vi "Process Calculation Results.vi"(8 "error in (no error)":errorcluster, 10 "Calculation Results":T1, 11 "CPU FFT Calculator in":refnum<class "CPU FFT Calculator.lvclass">) -> (0 "error out":errorcluster, 3 "CPU FFT Calculator out":refnum<class "CPU FFT Calculator.lvclass">)   [LabVIEW 2020, in "CPU FFT Calculator.lvlib" / "CPU FFT Calculator.lvclass"]
uses:
  CPU FFT Calculator.lvclass
  C:/Users/natan/Documents/G2CPU-Performance-Demo/Calculation Worker/Calculation Worker/Calculation Worker.lvclass
  C:/Program Files/National Instruments/LabVIEW 2026/vi.lib/ActorFramework/Actor/Actor.lvclass
  CPU Calculation Results.ctl
  CPU Metrics.ctl
  CPU FFT Calculator.lvclass/CPU FFT Calculator.ctl
  <vilib>/ActorFramework/Actor/Actor.lvclass/Actor.ctl
  Application Manager/Application Manager Messages/Update CPU UI Components Msg/Update CPU UI Components Msg.lvclass/Update CPU UI Components Msg.ctl
  <vilib>/ActorFramework/Message Enqueuer/Message Enqueuer.lvclass/Message Enqueuer.ctl
  Application Manager/Application Manager Messages/Update CPU Graph Msg/Update CPU Graph Msg.lvclass/Update CPU Graph Msg.ctl
  <vilib>/ActorFramework/Message Enqueuer/Enqueue.vi
  Application Manager/Application Manager Messages/Update CPU UI Components Msg/Update CPU UI Components Msg.lvclass
  C:/Program Files/National Instruments/LabVIEW 2026/vi.lib/ActorFramework/Message/Message.lvclass
  Application Manager/Application Manager Messages/Update CPU Graph Msg/Update CPU Graph Msg.lvclass
  <vilib>/ActorFramework/Message Priority Queue/Priority Enqueue.vi
  Simple UI/Simple UI/Simple UI.lvclass
  <vilib>/ActorFramework/Actor/Actor.lvclass
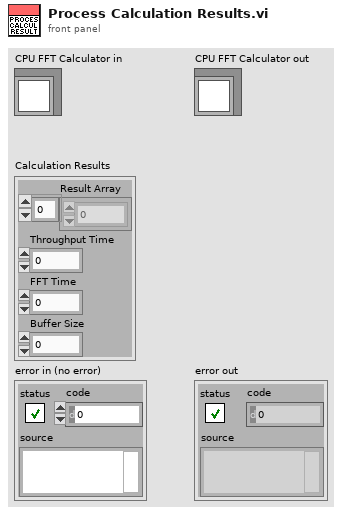
[diagram p1: front panel]
types:
  T1 = typedef "CPU FFT Calculator.lvlib/CPU FFT Calculator.lvclass/CPU Calculation Results.ctl" = cluster{"Result Array":sgl[], "Throughput Time":dbl, "FFT Time":dbl, "Buffer Size":i32}
  T2 = typedef "Simple UI.lvlib/Simple UI.lvclass/CPU Metrics.ctl" = cluster{"FFT Time":dbl, "Throughput":dbl, "Queue Depth":u64, "Elapsed Time":dbl}
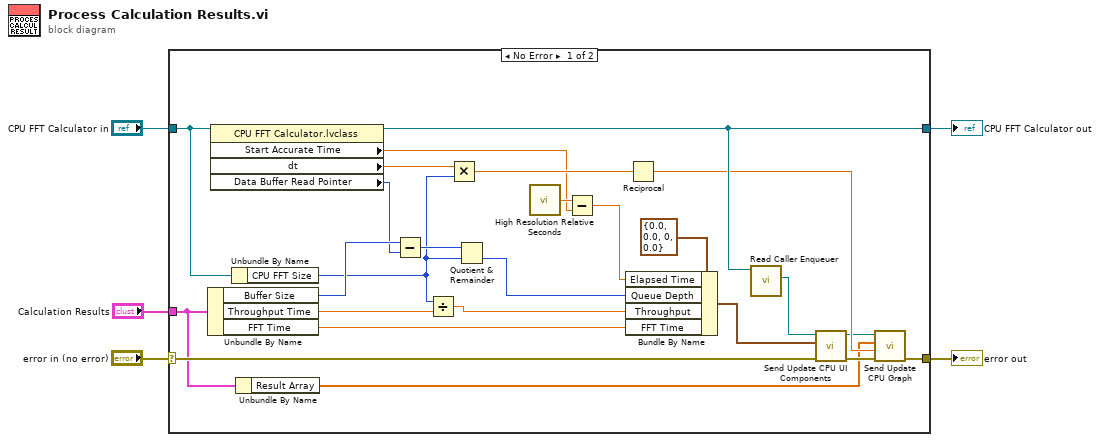
[diagram p0: block diagram]
diagram:
  n1 = case shown="No Error" "error in (no error)" {
    selector: "error in (no error)" -> [w24 w32]
    tunnel: [w16 w32] -> w4
    tunnel: [w22 w31] -> w2
    tunnel: "CPU FFT Calculator in" -> [w26 w31]
    tunnel: "Calculation Results" -> [w12 _]
    frame No Error {
      n2 = Unbundle By Name(w12) -> ("Buffer Size"=w21:i32, "Throughput Time"=w28:dbl, "FFT Time"=w29:dbl)
      n3 = property class="CPU FFT Calculator.lvclass"(reference=w26) -> (reference out=w22:refnum<class "CPU FFT Calculator.lvclass">, "Start Accurate Time"=w7:dbl, "dt"=w15:dbl, "Data Buffer Read Pointer"=w20:u64)  [unwired: 1 in, 1 out]
      n4 = Unbundle By Name(w26) -> ("CPU FFT Size"=w9:u64)
      n5 = Unbundle By Name(w12) -> ("Result Array"=w11:sgl[])
      n6 = Subtract(x=w21, y=w20) -> (x-y=w19:u64)
      n7 = Divide(x=w9, y=w28) -> (x/y=w27:dbl)
      n8 = Multiply(x=w15, y=w9) -> (x*y=w10:dbl)
      n9 = Quotient & Remainder(x=w19, y=w9) -> (floor(x/y)=w18:u64)  [unwired: 1 out]
      n10 = call <vilib>:"High Resolution Relative Seconds.vi"() -> ("relative seconds"=w8:dbl)
      n11 = Subtract(x=w8, y=w7) -> (x-y=w6:dbl)
      n12 = Bundle By Name(cluster=T2 {"FFT Time"=0.0, "Throughput"=0.0, "Queue Depth"=0, "Elapsed Time"=0.0} ("Cluster"), "Elapsed Time"=w6, "Queue Depth"=w18, "Throughput"=w27, "FFT Time"=w29) -> (w23:T2)
      n13 = Reciprocal(x=w10) -> (1/x=w14:dbl)
      n14 = call <vilib>:"Read Caller Enqueuer.vi"("Actor"=w22) -> ("Caller Enqueuer"=w25:refnum<class "Message Enqueuer.lvclass">)  [unwired: 10 in]
      n15 = call "Send Update CPU UI Components.vi"("error in (no error)"=w24, "CPU Metrics"=w23, "Message Enqueuer"=w25) -> ("error out"=w17:errorcluster, "Message Enqueuer out"=w13:refnum<class "Message Enqueuer.lvclass">)  [unwired: 7 in]
      n16 = call "Send Update CPU Graph.vi"("error in (no error)"=w17, "df"=w14, "Plot"=w11, "Message Enqueuer"=w13) -> ("error out"=w16:errorcluster)  [unwired: 6 in, 1 out]
    }
    frame Error {
    }
  }
  "error out" <- w4
  "CPU FFT Calculator out" <- w2
